vi "Get Logarithm Vertex.vi"(9 "Logarithm?":bool, 10 "Vertex Array In":sgl[](array[numeric]), 11 "Range In":cluster{"Max X":sgl, "Min X":sgl}) -> (2 "Vertex Array Out":sgl[](array[numeric]), 3 "Range Out":cluster{"Max":sgl, "Min":sgl})   [LabVIEW 2020, in "3D Plot.lvclass"]
uses:
  <vilib>/Math Plots/3D Math Plots/3D Plot/3D Plot/3D Plot.lvclass
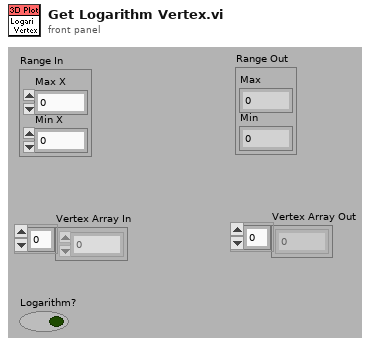
[diagram p1: front panel]
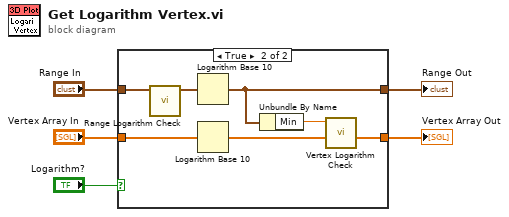
[diagram p0: block diagram]
diagram:
  n1 = case shown="True" "Logarithm?" {
    tunnel: "Vertex Array In" -> [w6 w14]
    tunnel: [w6 w10] -> w2
    tunnel: "Range In" -> [w7 w13]
    tunnel: [w7 w9] -> w3
    frame False {
    }
    frame True {
      n2 = call <vilib>:"Range Logarithm Check.vi"("Logarithm Range In"=w13) -> ("Logarithm Range Out"=w12:cluster{"Max":sgl, "Min":sgl})  [unwired: 10 out]
      n3 = Logarithm Base 10(1:w12) -> (0:w9:cluster{"Max":sgl, "Min":sgl})
      n4 = Logarithm Base 10(1:w14) -> (0:w11:sgl[])
      n5 = Unbundle By Name(w9) -> ("Min"=w8:sgl)
      n6 = call <vilib>:"Vertex Logarithm Check.vi"("Vertex Array In"=w11, "Range Min"=w8) -> ("Vertex Array Out"=w10:sgl[])  [unwired: 9 out]
    }
  }
  "Range Out" <- w3
  "Vertex Array Out" <- w2
